vi "Execute Subscription Policy.vi"(9 "Publish Time":timestamp, 10 "New Topic Value":variant, 11 "Subscription Policy":T1) -> (0 "error out (Unsubscribe?)":errorcluster)   [LabVIEW 2015]
doc: "This method decides whether or not to send or otherwise handle the new data value. The policy is set and maintained by the subscriber. The Topic Actor knows no policy details, it just passes the new value in. If there is a failure inside this method, the Topic Actor must assume the listener is no longer valid (dead/unrecoverable) and should delete it from the Subscriber list.\n\n<License>\nCopyright © 2017 Composed Systems, LLC | All rights reserved\nwww.composed.io\n\nAuthor: Ethan Stern <ethan.stern@composed.io>\n\nThis software is provided \"AS IS\" WITHOUT WARRANTIES, either express or implied, AND IS FOR EDUCATIONAL PURPOSES ONLY.\n</License>"
uses:
  BasicSubscription.lvclass
  ISubscriptionPolicy Reference.ctl
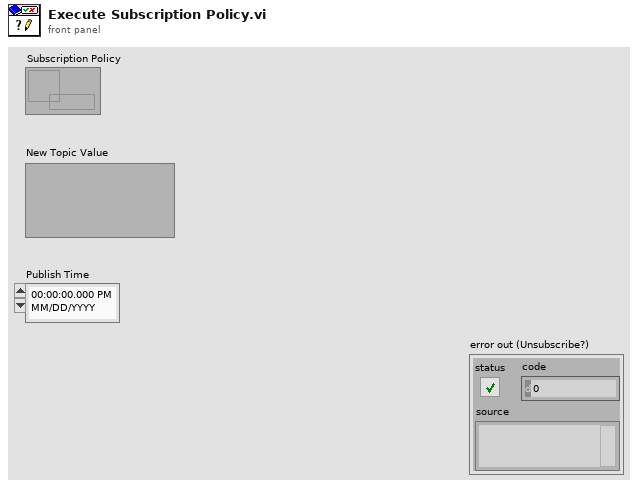
[diagram p1: front panel]
types:
  T1 = typedef "ISubscriptionPolicy Reference.ctl" = refnum<data-value>
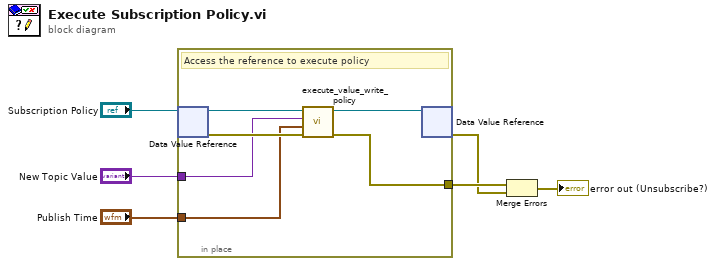
[diagram p0: block diagram]
diagram:
  n1 = in-place {
    in-place-border: "New Topic Value" -> [w9]
    in-place-border: "Publish Time" -> [w8]
    in-place-border: [w7] -> w3
    # "Access the reference to execute policy"
    n2 = in-place-dvr #1("Subscription Policy") -> (w12:refnum<class "BasicSubscription.lvclass">, w10:errorcluster)
    n3 = call-dynamic "execute_value_write_policy.vi"("error in (no error)"=w10, "Publish Time"=w8, "New Topic Value"=w9, "BasicSubscription In"=w12) -> ("error out"=w7:errorcluster, "BasicSubscription Out"=w11:refnum<class "BasicSubscription.lvclass">)  [unwired: 6 in]
    n4 = in-place-dvr #1(w11) -> (w2:errorcluster)  [unwired: 1 out]
  }
  n5 = Merge Errors(w3, w2) -> (→"error out (Unsubscribe?)":errorcluster)
